vi "Int2FXP_Quantize.vi"(8 "Output Bit resolution":i8=12, 9 "Input Bit resolution":i8=12, 10 "Multiplier":fxp<+,8,4>=10.0 format="%#_19g", 11 "Input (Int)":i16) -> (3 "Output (FXP)":fxp<+/-,25,5>)   [LabVIEW 2019, in "FPGA functions.lvlib"]
doc: "Convert 12-bit integer into Fixed Point (±16,5)\n\nSelect the appropriate quantization level"
uses:
  FPGA functions.lvlib
  <vilib>/Platform/TimedLoop/XDataNode/timing_clust.ctl
  <vilib>/Platform/TimedLoop/XDataNode/nitl_modes.ctl
  <vilib>/Platform/TimedLoop/XDataNode/wakeup.ctl
  <vilib>/rvi/Emulation/niFpgaSctlEmulationGetInTimedLoop.vi
  <vilib>/rvi/Emulation/niFpgaEmulationReportErrorSimple.vi
  <vilib>/rvi/Emulation/niFpgaGetClockAttributes.vi
  <vilib>/rvi/Emulation/niFpgaCriticalErrorInLSC.vi
  <vilib>/Platform/TimedLoop/XDataNode/XDataNode.xnode
  <vilib>/rvi/FXPMathLib/FxpMul/XNode/nifxpmath_Multiplier.xnode
  <vilib>/Platform/TimedLoop/XDataNode/XDNodeRunTimeDep.lvlib
  <vilib>/rvi/FXPMathLib/sim/FxpSim.dll
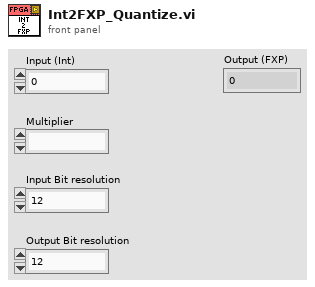
[diagram p1: front panel]
types:
  T1 = typedef "XDNodeRunTimeDep.lvlib/timing_clust.ctl" = cluster{"Expected End [f-1]":u64, "Actual End [f-1]":u64, "Finished Late? [f-1]":bool, "Expected End [i-1]":u64, "Actual End [i-1]":u64, "Finished Late? [i-1]":bool, "Expected Start [i]":u64, "Actual Start [i]":u64, "Expected Start [f]":u64, "Actual Start [f]":u64, "Source Name":string, "Structure Name":string, "Period":i64, "Deadline":i64, "Offset":i64, "Start":i64, "Priority":i32, "Timeout":i32, "Mode":T2, "Wakeup Reason":T3, "Error":errorcluster, "Source Type":string, "Secondary Source Type":string, "Global End Time":u64, "Global Start Time":u64, "Frame Duration":u64, "Iteration Duration":u64, "Assigned CPU":i32, "I/O Scan Engine Mode":u32}
  T2 = typedef "XDNodeRunTimeDep.lvlib/nitl_modes.ctl" = enum32{"No Change", "Process missed periods, maintain original phase", "Discard missed periods, maintain original phase", "Process missed periods, ignore original phase", "Discard missed periods, ignore original phase"}
  T3 = typedef "XDNodeRunTimeDep.lvlib/wakeup.ctl" = enum32{"Normal", "Aborted", "Asynchronous wakeup", "Timing source error", "Timed loop error", "Timeout"}
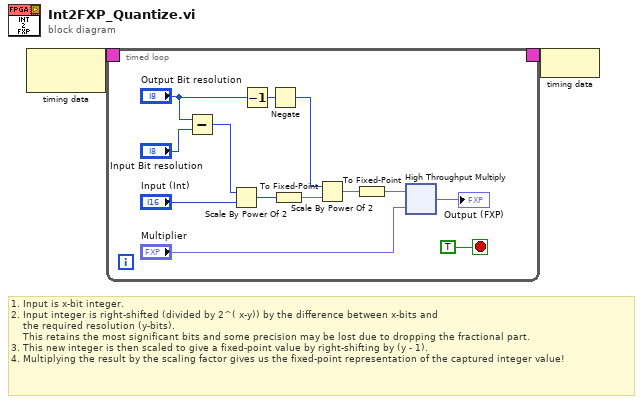
[diagram p0: block diagram]
diagram:
  # "1. Input is x-bit integer. \n2. Input integer is right-shifted (divided by 2^( x-y)) by the difference between x-bits and \n    the required resolution (y-bits).\n    This retains the most significant bits and some precision may be lost due to dropping the fractional part.\n3. This new integer is then scaled to give a fixed-point value by right-shifting by (y - 1).\n4. Multiplying the result by the scaling factor gives us the fixed-point representation of the captured integer value!"
  n1 = node-c288() -> (w2:T1)  [unwired: 1 in]
  n2 = timed-loop {
    timing: w2 -> [_]
    timing-out: [_] -> w1
    stop <- TRUE stop-if-true
    n3 = Subtract(x="Output Bit resolution", y="Input Bit resolution") -> (x-y=w7:i8)
    n4 = Scale By Power Of 2(n=w7, x="Input (Int)") -> (x*2^n=w6:i16)
    n5 = Decrement(x="Output Bit resolution") -> (x-1=w5:i8)
    n6 = Negate(x=w5) -> (-x=w3:i8)
    n7 = To Fixed-Point(number=w6) -> (fixed-point=w15:fxp<+/-,32,16>)  [unwired: 1 in]
    n8 = Scale By Power Of 2(n=w3, x=w15) -> (x*2^n=w13:fxp<+/-,32,16>)
    n9 = To Fixed-Point(number=w13) -> (fixed-point=w12:fxp<+/-,18,5>)  [unwired: 1 in]
    n10 = xnode "High Throughput Multiply"("x"=w12, "y"="Multiplier") -> ("x*y"=→"Output (FXP)":fxp<+/-,25,5>)
  }
  n11 = node-c288(w1) -> ()
